vi "Read User Interface Object.vi"(8 "error in (no error)":errorcluster, 11 "UI Controller in":refnum<class "Controller.lvclass">) -> (0 "error out":errorcluster, 2 "UI.lvclass":refnum<class "UI.lvclass">, 3 "UI Controller out":refnum<class "Controller.lvclass">)   [LabVIEW 2016, in "Controller Actor.lvlib" / "Controller.lvclass"]
uses:
  Controller.lvclass
  User Interface/UI.lvclass
  Controller.lvclass/Controller.ctl
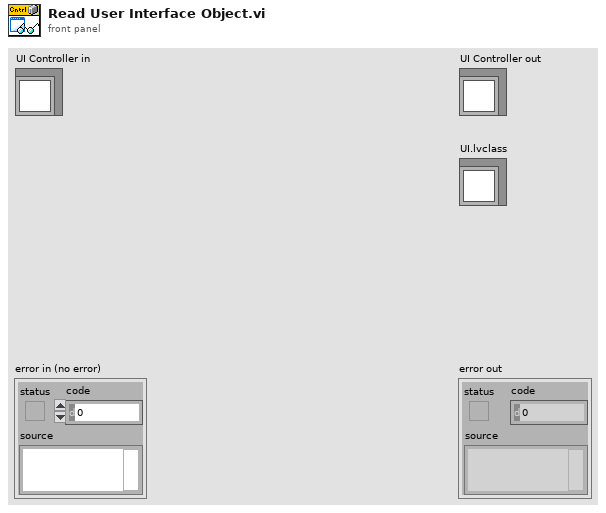
[diagram p1: front panel]
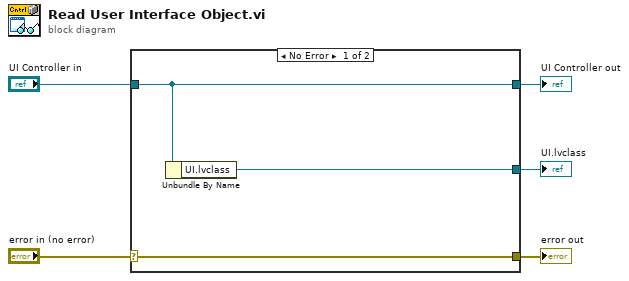
[diagram p0: block diagram]
diagram:
  n1 = case shown="No Error" "error in (no error)" {
    selector: "error in (no error)" -> [w8 w9]
    tunnel: [w8 w9] -> w4
    tunnel: [w7 w10] -> w2
    tunnel: "UI Controller in" -> [w7 w10]
    tunnel: [w6 _] -> w1
    frame No Error {
      n2 = Unbundle By Name(w7) -> ("UI.lvclass"=w6:refnum<class "UI.lvclass">)
    }
    frame Error {
    }
  }
  "error out" <- w4
  "UI Controller out" <- w2
  "UI.lvclass" <- w1
